vi "shoot.vi"(6 "speedScaling":dbl=1.0, 7 "shot delay":dbl=0.5, 8 "offset":dbl=1.05, 9 "Button 1":bool, 10 "axis 3 (throttle)":dbl, 11 "speedFactor":dbl=1.05) -> ()   [LabVIEW 2011]
uses:
  <vilib>/Rock Robotics/WPI/Solenoid/WPI_SolenoidValue.ctl
  <vilib>/Rock Robotics/WPI/Solenoid/WPI_SolenoidSetEnum.vi
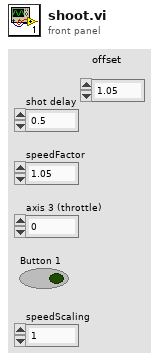
[diagram p1: front panel]
types:
  T1 = typedef "WPI_SolenoidDevRef.ctl" = cluster{"DevStatus":errorcluster, "Solenoid Module":T2, "Forward Solenoid Channel":T3, "Reverse Solenoid Channel":T3}
  T2 = typedef "FPGA_TypedefSolenoidModule.ctl" = enum16{"Solenoid Module 1", "Solenoid Module 2"}
  T3 = typedef "WPI_SolenoidChannel.ctl" = enum8{"Solenoid 1", "Solenoid 2", "Solenoid 3", "Solenoid 4", "Solenoid 5", "Solenoid 6", "Solenoid 7", "Solenoid 8", "Invalid"}
  T4 = typedef "WPI_RobotDriveDevRef.ctl" = cluster{"DevStatus":errorcluster, "Motors[]":T5[], "Square Inputs":bool, "Max Output":dbl, "Isochronous":bool}
  T5 = typedef "WPI_MotorControlDeviceRef.ctl" = cluster{"DeviceStatus":errorcluster, "Type":enum16{"PWM", "CAN"}, "PWM":cluster{"Digital Module":T6, "PWM Channel":T7, "DeadBand":T8}, "CAN":cluster{"Device Number":u8, "Control Mode":T9, "Semaphore":T10, "Max Vout":dbl}, "Invert":bool, "TransformRef":T11, "InvTransformRef":T11}
  T6 = typedef "FPGA_TypedefDigitalModule.ctl" = enum16{"Digital Module 1", "Digital Module 2"}
  T7 = typedef "FPGA_DIOPWMChannel.ctl" = enum8{"PWM 1", "PWM 2", "PWM 3", "PWM 4", "PWM 5", "PWM 6", "PWM 7", "PWM 8", "PWM 9", "PWM 10", "Invalid"}
  T8 = typedef "WPI_PWMDeadband.ctl" = cluster{"Name":string, "maxPositivePwm":i32, "minPositivePwm":i32, "centerPwm":i32, "maxNegativePwm":i32, "minNegativePwm":i32, "angularRange":u16}
  T9 = typedef "WPI_CANJaguar_ControlMode.ctl" = enum8{"Percent VBus", "Current", "Speed", "Position", "Voltage"}
  T10 = typedef "Semaphore RefNum" = refnum<k1>
  T11 = typedef "WPI_PWMTransform_ConPane.ctl" = refnum<vi>
  T12 = typedef "WPI_SolenoidValue.ctl" = enum16{"Off", "On", "Forward", "Reverse"}
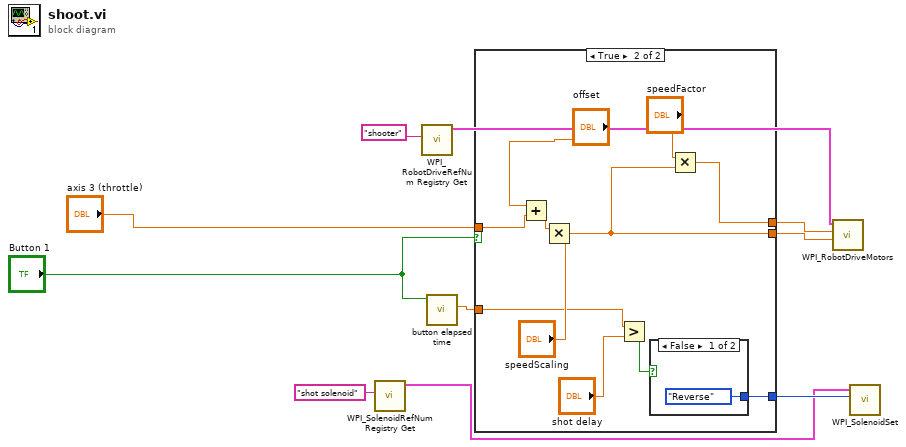
[diagram p0: block diagram]
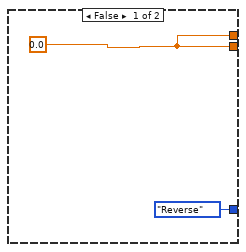
[diagram p2: hidden frame]
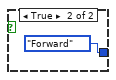
[diagram p3: hidden frame]
diagram:
  n1 = call <vilib>:"WPI_SolenoidRefNum Registry Get.vi"("refnum name"="shot solenoid") -> ("SolenoidDevRef"=w9:T1)  [unwired: 9 in, 1 out]
  n2 = call <vilib>:"WPI_RobotDriveRefNum Registry Get.vi"("refnum name"="shooter") -> ("RobotDriveDevRef"=w2:T4)  [unwired: 1 in, 9 out]
  n3 = call "button elapsed time.vi"("Button"="Button 1") -> ("Elapsed time"=w7:dbl)  [unwired: 10 in]
  n4 = case shown="True" "Button 1" {
    tunnel: "axis 3 (throttle)" -> [_ w15]
    tunnel: [w12 w21] -> w4
    tunnel: [w12 w22] -> w5
    tunnel: w7 -> [_ w19]
    tunnel: [WPI_SolenoidValue."Reverse" ("Value") w17] -> w10
    frame False {
      w12 = 0.0 ("RightSpeed")
    }
    frame True {
      n5 = Add(x="offset", y=w15) -> (x+y=w14:dbl)
      n6 = Multiply(x=w14, y="speedScaling") -> (x*y=w21:dbl)
      n7 = Greater?(x=w19, y="shot delay") -> (0:w16:bool)
      n8 = case shown="False" w16 {
        tunnel: [WPI_SolenoidValue."Reverse" ("Value") WPI_SolenoidValue."Forward" ("Value")] -> w17
        frame False {
        }
        frame True {
        }
      }
      n9 = Multiply(x="speedFactor", y=w21) -> (x*y=w22:dbl)
    }
  }
  n10 = call <vilib>:"WPI_RobotDriveMotors.vi"("RightSpeed"=w4, "LeftSpeed"=w5, "RobotDriveDevRef"=w2) -> ()  [unwired: 7 in, 2 out]
  n11 = call-poly <vilib>:"WPI_SolenoidSet.vi"("Value"=w10, "SolenoidDevRef"=w9) -> ()  [unwired: 8 in, 2 out]
